vi "15_Waveform Chart.vi"() -> ()   [LabVIEW 2018]
panel:
  in  "stop":bool
  out "Waveform Chart":dbl(graph)
  out "x+y":dbl
  # "Procedure:\n1.\tOpen NI LabVIEW 2018 and press <Ctrl_N> to open a blank VI.\n2.\tPress <Ctrl_T> to tile front panel and block diagram windows.\n3.\tPull up the Functions Palette by right_clicking on the white space on the LabVIEW block diagram window.\n4.\tSelect Programming>>Structures>>For Loop and drop in the Block Diagram.\n5.\tRight click on count terminal (N) of loop and select create constant.\n5.\tSelect Programming>>Numeric>>Add and place it inside the loop in the Block Diagram.\n6.\tRight click any one of the input terminal and select create constant and set it to 1.\n7.\tFor Time Delay select Programming>>Timing>>Wait(ms) and give 100 ms delay.\n8.\tFor the feedback node take the output from the adder and connect it to the other input.\n9.\tSelect indicator from Express>>Numeric Indicator and place in the front panel.\n10.\tPlace waveform chart in the front panel f rom Express>>Graph indicators.\n11.\tConnect indicator and chart to the output of adder in the Block Diagram.\n12.\tNow Run the VI and observe the numeric data and the Chart for while Loop.\n13.\tSave the file with extension \".vi\", a virtual instrument."
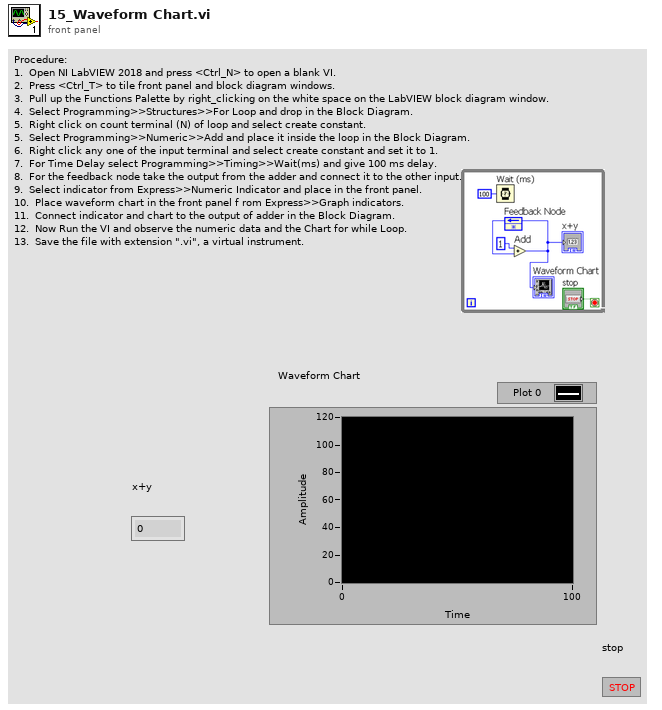
[diagram p1: front panel]
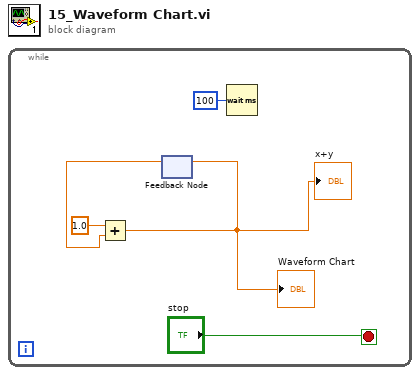
[diagram p0: block diagram]
diagram:
  n1 = while {
    stop <- "stop" stop-if-true
    n2 = feedback #1() -> (w2:dbl)  [unwired: 1 in]
    n3 = Add(x=1.0, y=w2) -> (x+y=w3:dbl)
    "x+y" <- w3
    "Waveform Chart" <- w3
    n4 = feedback-in #1(w3) -> ()
    n5 = Wait (ms)(milliseconds to wait=u32 100) -> ()  [unwired: 1 out]
  }
